vi "Dresser DXD Utility Default Instrument Setup.vi"(0 "VISA session":refnum<visa-resource-name>, 11 "Error In (no error)":errorcluster) -> (4 "dup VISA session":refnum<visa-resource-name>, 15 "Error Out":errorcluster)   [LabVIEW 2015]
doc: "This Utility VI is part of the standard National Instruments driver requirements and would send a default command string to the instrument whenever a new VISA session is opened if the command were supported. This VI is intended to be used as a subVI for the Dresser DXD Initialize and Dresser DXD Reset VI's. Altering this VI could cause these two VI's to operate incorrectly. If a default command is to be implemented, show the true case on the diagram, right click on the case structure and select remove case structure, and enter the command string.\n\nWritten by:\nBLOOMY CONTROLS, INC\nWINDSOR, CT 06095, USA\n860-298-9925\nwww.bloomy.com\nV2.0.0\nMay, 2002"
panel:
  in  "Case Constant\n(See Context Help)":bool
  # "For instructions on the use of this VI, press Ctrl+H to display the help window and move the mouse over the icon, controls, and indicators"
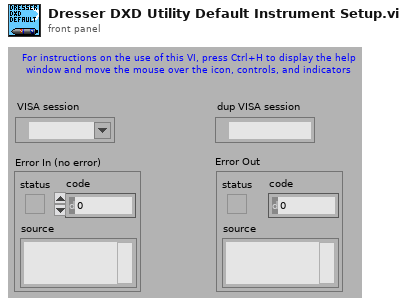
[diagram p1: front panel]
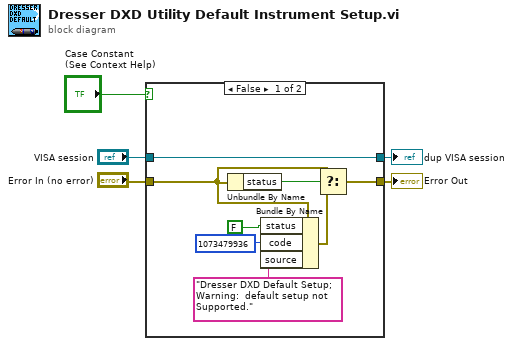
[diagram p0: block diagram]
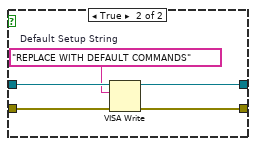
[diagram p2: hidden frame]
diagram:
  n1 = case shown="False" "Case Constant\n(See Context Help)" {
    tunnel: "VISA session" -> [w13 w18]
    tunnel: "Error In (no error)" -> [w7 w17]
    tunnel: [w13 w16] -> w3
    tunnel: [w6 w15] -> w2
    frame False {
      n2 = Unbundle By Name(w7) -> ("status"=w9:bool)
      n3 = Bundle By Name(cluster=w7, "status"=FALSE, "code"=1073479936, "source"="Dresser DXD Default Setup; Warning:  default setup not Supported.") -> (w8:errorcluster)
      n4 = Select(t=w7, s=w9, f=w8) -> (s? t:f=w6:errorcluster)
    }
    frame True {
      w14 = "REPLACE WITH DEFAULT COMMANDS"  # Default Setup String
      n5 = VISA Write(VISA resource name=w18, write buffer=w14, error in (no error)=w17) -> (VISA resource name out=w16:refnum<visa-resource-name>, error out=w15:errorcluster)  [unwired: 1 out]
    }
  }
  "Error Out" <- w2
  "dup VISA session" <- w3
